vi "Analog_Output.vi"(8 "error in":errorcluster caption="entrée d'erreur") -> (0 "error out":errorcluster caption="sortie d'erreur")   [LabVIEW 2026]
uses:
  <userlib>/LV-Link3/PolySubVIs/DtCreateAoutChan.vi
  <userlib>/LV-Link3/PolySubVIs/DtOLWriteSingle.vi
panel:
  in  "Channel #":string="1"
  in  "Output voltage":dbl(slide) min=-10.0 max=10.0 step=0.1 scale=-10.0..10.0
  in  "stop":bool
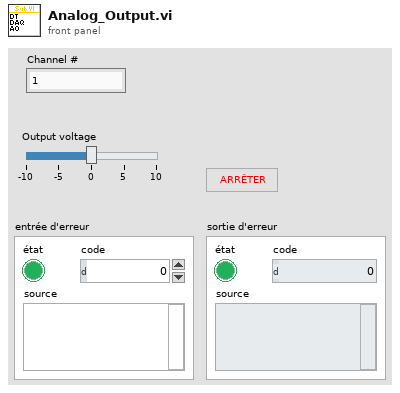
[diagram p1: front panel]
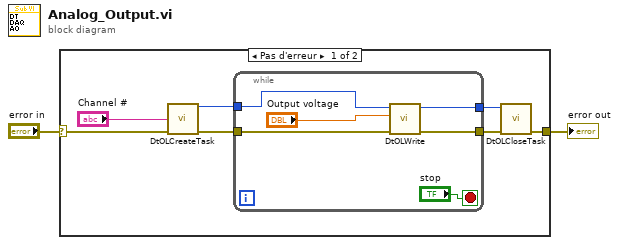
[diagram p0: block diagram]
diagram:
  n1 = case shown="Pas d'erreur" "error in" {
    selector: "error in" -> [w7 w16]
    tunnel: [w8 w16] -> w2
    frame No Error {
      n2 = call-poly <userlib>:"DtOLCreateTask.vi"("Channel"="Channel #", "error in (no error)"=w7) -> ("Task out"=w5:i32, "error out"=w6:errorcluster)  [unwired: 11 in, 1 out]
      n3 = while {
        tunnel: w6 -> [w12]
        tunnel: w5 -> [w13]
        tunnel: [w11] -> w4
        tunnel: [w14] -> w9
        stop <- "stop" stop-if-true
        n4 = call-poly <userlib>:"DtOLWrite.vi"("error in (no error)"=w12, "Data In"="Output voltage", "Task in"=w13) -> ("error out"=w11:errorcluster, "Task out"=w14:i32)  [unwired: 7 in]
      }
      n5 = call <userlib>:"DtOLCloseTask.vi"("Error in"=w4, "Task in"=w9) -> ("Error Out"=w8:errorcluster)  [unwired: 9 in]
    }
    frame Error {
    }
  }
  "error out" <- w2
